vi "test.Create.OrderExecuted.vi"(11 "OrderExecuted.Parameters":T1={"Time Offset"=447000, "Order Id"="ORID0001", "Executed Quantity"=20000, "Execution Id"="AAPL"}) -> (3 "Passed":bool)   [LabVIEW 2022 SP3]
uses:
  OrderExecuted/OrderExecuted.Parameters.ctl
  OrderExecuted/OrderExecuted.lvclass
panel:
  out "x = y?":bool[](array[boolean])
  out "Python.Bytes.Out":u8[](array[numeric]) format="%.0x"
  out "LabVIEW.Bytes.Out":u8[](array[numeric]) format="%.0x"
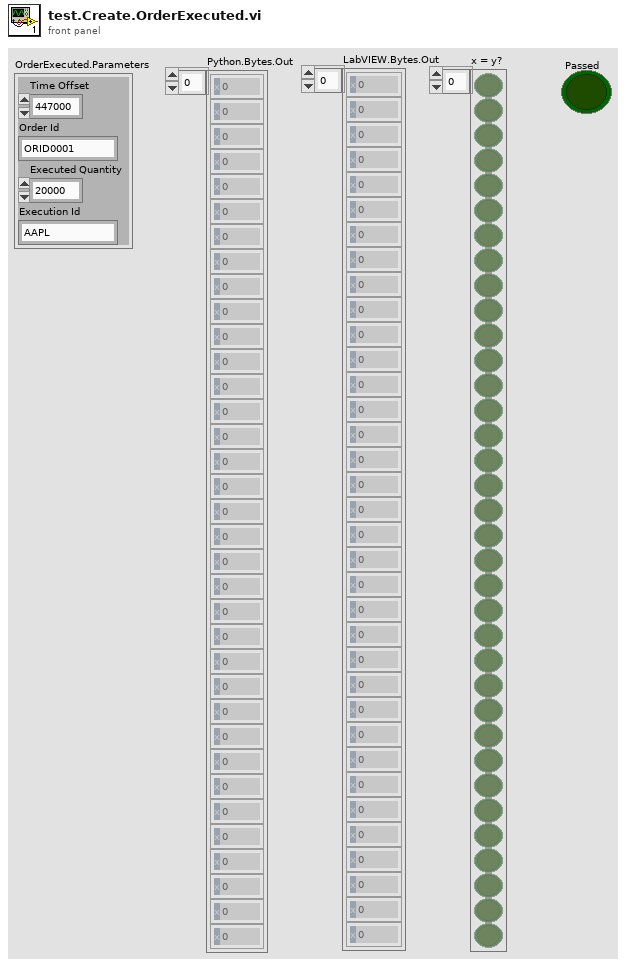
[diagram p1: front panel]
types:
  T1 = typedef "OrderExecuted.lvclass/OrderExecuted.Parameters.ctl" = cluster{"Time Offset":u32, "Order Id":string, "Executed Quantity":u32, "Execution Id":string}
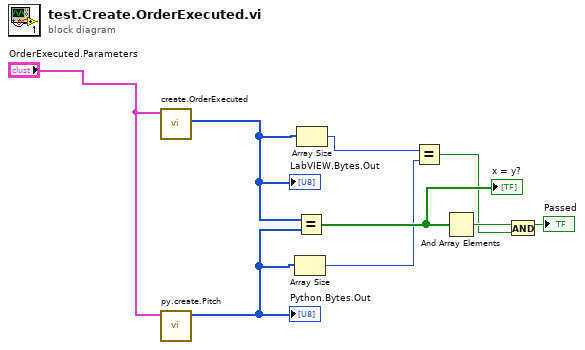
[diagram p0: block diagram]
diagram:
  n1 = call "create.OrderExecuted.vi"("OrderExecuted.Parameters"="OrderExecuted.Parameters") -> ("Bytes.Out"=w6:u8[])  [unwired: 10 in]
  "LabVIEW.Bytes.Out" <- w6
  n2 = call "py.create.Pitch.vi"("Parameters"="OrderExecuted.Parameters") -> ("bytes"=w5:u8[])  [unwired: 9 in, 1 out]
  "Python.Bytes.Out" <- w5
  n3 = Array Size(array=w5) -> (size(s)=w3:i32)
  n4 = Equal?(x=w6, y=w5) -> (x = y?=w9:bool[])
  "x = y?" <- w9
  n5 = Array Size(array=w6) -> (size(s)=w4:i32)
  n6 = Equal?(x=w4, y=w3) -> (x = y?=w1:bool)
  n7 = And Array Elements(Boolean array=w9) -> (logical AND=w8:bool)
  n8 = And(x=w8, y=w1) -> (x .and. y?=→"Passed":bool)
